vi "Handle Error.vi"(8 "error in (no error)":errorcluster, 11 "Field Drawer in":refnum<class "Field Drawer.lvclass">) -> (0 "error out":errorcluster, 2 "stop actor?":bool=TRUE, 3 "Field Drawer out":refnum<class "Field Drawer.lvclass">)   [LabVIEW 2022 SP3, in "Vision.lvlib" / "Field Drawer.lvlib" / "Field Drawer.lvclass"]
doc: "(<B>Filename</B>: Actor Framework.lvlib:Actor.lvclass:Handle Error.vi)\n\nDefines how the actor handles an error that occurred while processing a message.\n\nBy default, this method does nothing except stop the actor. This method also treats error code 43 (coming from <B>error in</B>) as a sign that the actor shut down normally. In this situation, the Handle Error method does not return the error on <B>error out</B>, meaning the actor's caller will not receive it. All other error codes will be returned on <B>error out</B>.\n\nA descendant class may override this method to change this behavior."
uses:
  Field Drawer.lvclass
  Field Drawer.lvclass/Field Drawer.ctl
  <vilib>/ActorFramework/Actor/Actor.lvclass
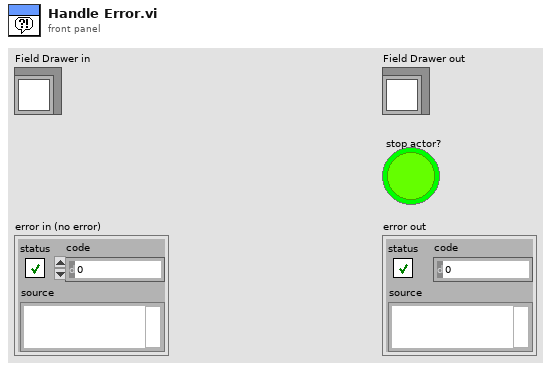
[diagram p1: front panel]
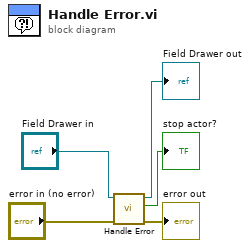
[diagram p0: block diagram]
diagram:
  n1 = call-parent "Handle Error.vi"("error in (no error)"="error in (no error)", "Actor in"="Field Drawer in") -> ("error out"=→"error out":errorcluster, "stop actor?"=→"stop actor?":bool, "Actor out"=→"Field Drawer out":refnum<class "Field Drawer.lvclass">)  [unwired: 7 in]
